vi "Get BYU ID.vi"(11 "REFERENCES":T1) -> (3 "USER/ITEM DATA TRANSFER":T2(array[cluster]))   [LabVIEW 2019]
uses:
  Controls/References Cluster.ctl
  Controls/Custom Calendar/Custom Calendar.xctl
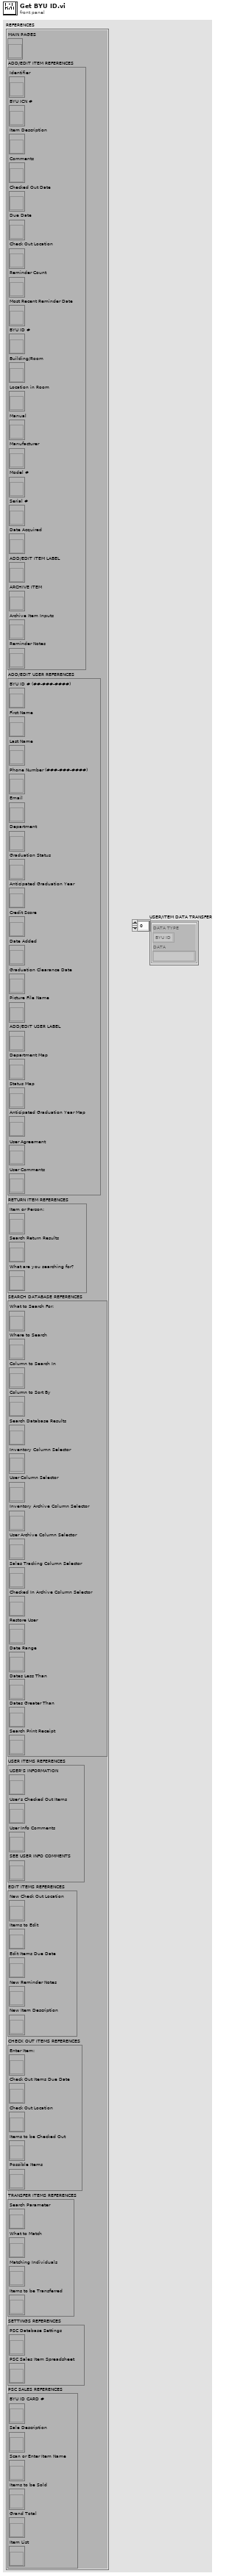
[diagram p1: front panel]
types:
  T1 = typedef "References Cluster.ctl" = cluster{"MAIN PAGES":refnum<vi>, "ADD/EDIT ITEM REFERENCES":cluster{"Identifier":refnum<vi>, "BYU ICN #":refnum<vi>, "Item Description":refnum<vi>, "Comments":refnum<vi>, "Checked Out Date":refnum<vi>, "Due Date":refnum<vi>, "Check Out Location":refnum<vi>, "Reminder Count":refnum<vi>, "Most Recent Reminder Date":refnum<vi>, "BYU ID #":refnum<vi>, "Building/Room":refnum<vi>, "Location in Room":refnum<vi>, "Manual":refnum<vi>, "Manufacturer":refnum<vi>, "Model #":refnum<vi>, "Serial #":refnum<vi>, "Date Acquired":refnum<vi>, "ADD/EDIT ITEM LABEL":refnum<vi>, "ARCHIVE ITEM":refnum<vi>, "Archive Item Inputs":refnum<vi>, "Reminder Notes":refnum<vi>}, "ADD/EDIT USER REFERENCES":cluster{"BYU ID # (##-###-####)":refnum<vi>, "First Name":refnum<vi>, "Last Name":refnum<vi>, "Phone Number (###-###-####)":refnum<vi>, "Email":refnum<vi>, "Department":refnum<vi>, "Graduation Status":refnum<vi>, "Anticipated Graduation Year":refnum<vi>, "Credit Score":refnum<vi>, "Date Added":refnum<vi>, "Graduation Clearance Date":refnum<vi>, "Picture File Name":refnum<vi>, "ADD/EDIT USER LABEL":refnum<vi>, "Department Map":refnum<vi>, "Status Map":refnum<vi>, "Anticipated Graduation Year Map":refnum<vi>, "User Agreement":refnum<vi>, "User Comments":refnum<vi>}, "RETURN ITEM REFERENCES":cluster{"Item or Person:":refnum<vi>, "Search Return Results":refnum<vi>, "What are you searching for?":refnum<vi>}, "SEARCH DATABASE REFERENCES":cluster{"What to Search For:":refnum<vi>, "Where to Search":refnum<vi>, "Column to Search In":refnum<vi>, "Column to Sort By":refnum<vi>, "Search Database Results":refnum<vi>, "Inventory Column Selector":refnum<vi>, "User Column Selector":refnum<vi>, "Inventory Archive Column Selector":refnum<vi>, "User Archive Column Selector":refnum<vi>, "Sales Tracking Column Selector":refnum<vi>, "Checked In Archive Column Selector":refnum<vi>, "Restore User":refnum<vi>, "Date Range":refnum<vi>, "Dates Less Than":refnum<vi>, "Dates Greater Than":refnum<vi>, "Search Print Receipt":refnum<vi>}, "USER ITEMS REFERENCES":cluster{"USER'S INFORMATION":refnum<vi>, "User's Checked Out Items":refnum<vi>, "User Info Comments":refnum<vi>, "SEE USER INFO COMMENTS":refnum<vi>}, "EDIT ITEMS REFERENCES":cluster{"New Check Out Location":refnum<vi>, "Items to Edit":refnum<vi>, "Edit Items Due Date":refnum<vi>, "New Reminder Notes":refnum<vi>, "New Item Description":refnum<vi>}, "CHECK OUT ITEMS REFERENCES":cluster{"Enter Item:":refnum<vi>, "Check Out Items Due Date":refnum<vi>, "Check Out Location":refnum<vi>, "Items to be Checked Out":refnum<vi>, "Possible Items":refnum<vi>}, "TRANSFER ITEMS REFERENCES":cluster{"Search Parameter":refnum<vi>, "What to Match":refnum<vi>, "Matching Individuals":refnum<vi>, "Items to be Transferred":refnum<vi>}, "SETTINGS REFERENCES":cluster{"PSC Database Settings":refnum<vi>, "PSC Sales Item Spreadsheet":refnum<vi>}, "PSC SALES REFERENCES":cluster{"BYU ID CARD #":refnum<vi>, "Sale Description":refnum<vi>, "Scan or Enter Item Name":refnum<vi>, "Items to be Sold":refnum<vi>, "Grand Total":refnum<vi>, "Item List":refnum<vi>}}
  T2 = cluster{"DATA TYPE":enum16{"BYU ID", "ME#/IDENTIFIER", "BYU ICN"}, "DATA":string}[]
  T3 = cluster{"DATA TYPE":enum16{"BYU ID", "ME#/IDENTIFIER", "BYU ICN"}, "DATA":string}
  T4 = cluster{"USER'S INFORMATION":refnum<vi>, "User's Checked Out Items":refnum<vi>, "User Info Comments":refnum<vi>, "SEE USER INFO COMMENTS":refnum<vi>}
  T5 = typedef "IMAQ Image.ctl" = refnum<image>
  T6 = cluster{"BYU ID #":string, "First Name":string, "Last Name":string, "Phone":string, "Email":string, "Department":string, "Status":string, "Grad Year":string, "Date Added":string, "Grad Clearance Date":string, "Credit Score":string, "User Items Photo":T5}
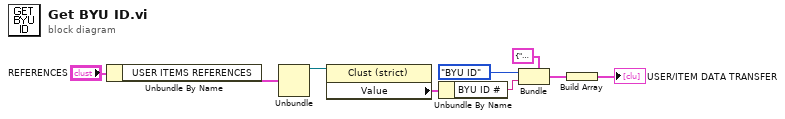
[diagram p0: block diagram]
diagram:
  n1 = Unbundle By Name("REFERENCES") -> ("USER ITEMS REFERENCES"=w1:T4)
  n2 = Unbundle(w1) -> ("USER'S INFORMATION"=w9:refnum<vi>)  [unwired: 3 out]
  n3 = property class="Clust (strict)"(reference=w9) -> ("Value"=w8:T6)  [unwired: 1 in, 2 out]
  n4 = Unbundle By Name(w8) -> ("BYU ID #"=w5:string)
  n5 = Bundle(cluster=T3 {"DATA TYPE"=enum."BYU ID", "DATA"=""} ("USER/ITEM DATA TRANSFER"), "DATA TYPE"=enum16{"BYU ID", "ME#/IDENTIFIER", "BYU ICN"}."BYU ID", "DATA"=w5) -> (w4:T3)
  n6 = Build Array(w4) -> (→"USER/ITEM DATA TRANSFER":T2)
